vi "get_shutter.vi"(8 "error in (no error)":errorcluster, 11 "LightSourceMH110124MaiTai in":refnum<class "LightSourceMH110124MaiTai.lvclass">) -> (0 "error out":errorcluster, 2 "shutter open out?":bool, 3 "LightSourceMH110124MaiTai out":refnum<class "LightSourceMH110124MaiTai.lvclass">)   [LabVIEW 2010, in "LightSourceMH110124MaiTai.lvclass"]
uses:
  LightSourceMH110124MaiTai.lvclass
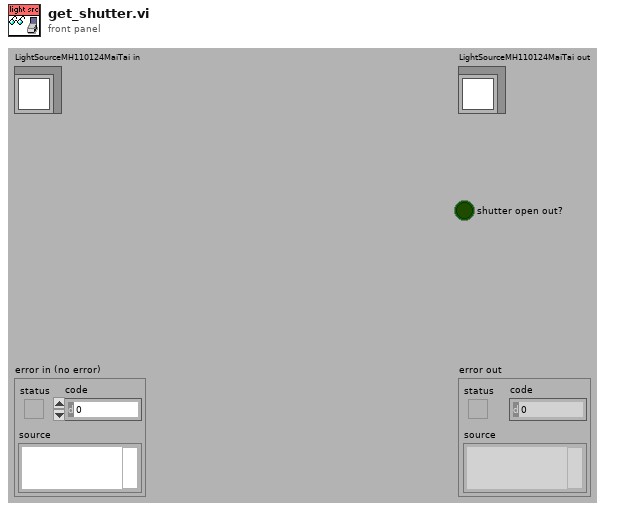
[diagram p1: front panel]
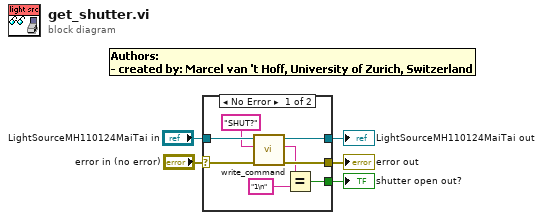
[diagram p0: block diagram]
diagram:
  n1 = case shown="No Error" "error in (no error)" {
    selector: "error in (no error)" -> [w11 w14]
    tunnel: [w10 w14] -> w4
    tunnel: [w12 w15] -> w3
    tunnel: "LightSourceMH110124MaiTai in" -> [w13 w15]
    tunnel: [w6 _] -> w1
    frame No Error {
      n2 = call-dynamic "write_command.vi"("error in (no error)"=w11, "string to write"="SHUT?", "LightSourceMH110124MaiTai in"=w13) -> ("error out"=w10:errorcluster, "read string"=w7:string, "LightSourceMH110124MaiTai out"=w12:refnum<class "LightSourceMH110124MaiTai.lvclass">)  [unwired: 6 in]
      n3 = Equal?(x=w7, y="1\n") -> (x = y?=w6:bool)
    }
    frame Error {
    }
  }
  "error out" <- w4
  "LightSourceMH110124MaiTai out" <- w3
  "shutter open out?" <- w1
